vi "Manage TCP Link Reference.vi"() -> ()   [LabVIEW 2016, in "Assert API Components.lvlib" / "Log Assert Core.lvlib"]
uses:
  Log Assert Core.lvlib
panel:
  out "error out":errorcluster
  in  "error in (no error)":errorcluster
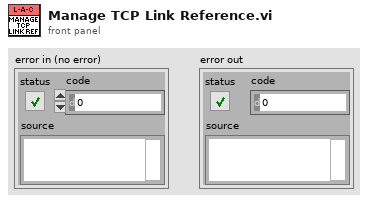
[diagram p1: front panel]
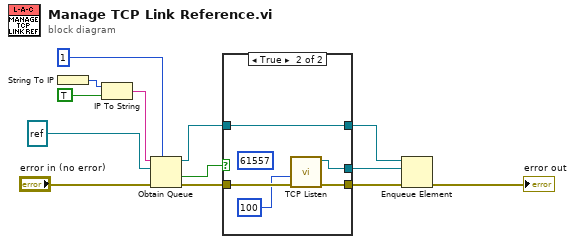
[diagram p0: block diagram]
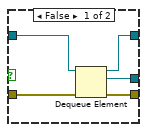
[diagram p2: hidden frame]
diagram:
  n1 = String To IP() -> (0:w10:u32)  [unwired: 1 in]
  n2 = IP To String(1:TRUE ("dot notation? (F)"), 2:w10) -> (0:w8:string)
  n3 = Obtain Queue(max queue size (-1, unlimited)=1, name (unnamed)=w8, element data type=refnum<k5> refnum ("connection ID"), error in (no error)="error in (no error)") -> (queue out=w6:refnum<queue>, created new?=w7:bool, error out=w11:errorcluster)  [unwired: 1 in]
  n4 = case shown="True" w7 {
    tunnel: [w15 w19] -> w3
    tunnel: [w14 w23] -> w12
    tunnel: w11 -> [w18 w22]
    tunnel: w6 -> [w17 w21]
    tunnel: [w16 w21] -> w4
    frame False {
      n5 = Dequeue Element(queue=w17, error in (no error)=w18) -> (queue out=w16:refnum<queue>, element=w15:refnum<k5>, error out=w14:errorcluster)  [unwired: 1 in, 1 out]
    }
    frame True {
      (unwired) u16 61557 ("local port")
      n6 = call <vilib>:"TCP Listen.vi"("error in (no error)"=w22, "timeout ms (wait forever: -1)"=100 ("timeout ms (25000)")) -> ("error out"=w23:errorcluster, "connection ID"=w19:refnum<k5>)  [unwired: 5 in, 3 out]
    }
  }
  n7 = Enqueue Element(queue=w4, element=w3, error in (no error)=w12) -> (error out=→"error out":errorcluster)  [unwired: 1 in, 2 out]
